vi "cam take photo-box.vi"(7 "error in":errorcluster) -> (20 "Image Out":T2(plugin-control), 22 "Session Out":T1, 27 "error out":errorcluster)   [LabVIEW 2019]
doc: "Creates, and edits acquisitions using the NI Vision Acquisition Express VI.\n\nThe NI Vision Acquisition Wizard is launched by placing the Express VI on the block diagram. Select an acquisition source and configure an acquisition using NI-IMAQ, NI-IMAQdx, or simulate an acquisition by reading an AVI or image files from a folder. After an acquisition is configured, select controls and indicators to be able to programmatically set in LabVIEW. Double-click the Vision Acquisition Express VI to edit the acquisition.\n\nNote: Any images created by the Express VI need to be disposed after use. Use the IMAQ Dispose.vi to cleanup the images output by the Express VI when they are no longer needed."
uses:
  <vilib>/userDefined/High Color/IMAQdx.ctl
  <vilib>/vision/driver/NI_Vision_Acquisition_Software.lvlib
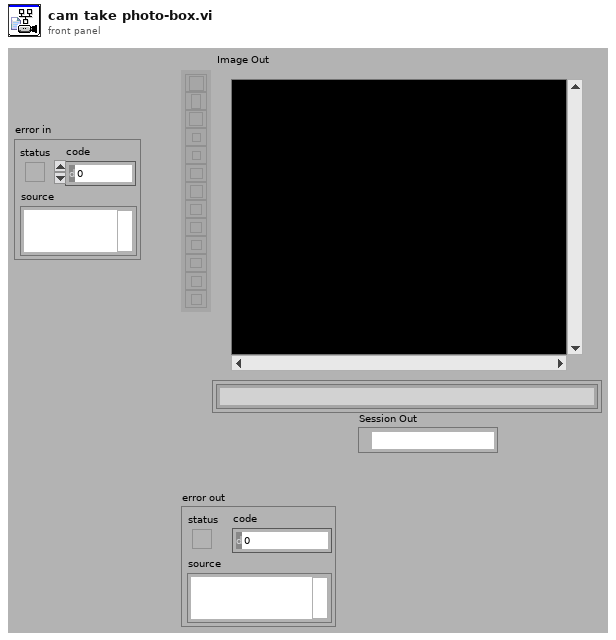
[diagram p1: front panel]
types:
  T1 = typedef "IMAQdx.ctl" = refnum<k21>
  T2 = typedef "IMAQ Image.ctl" = refnum<image>
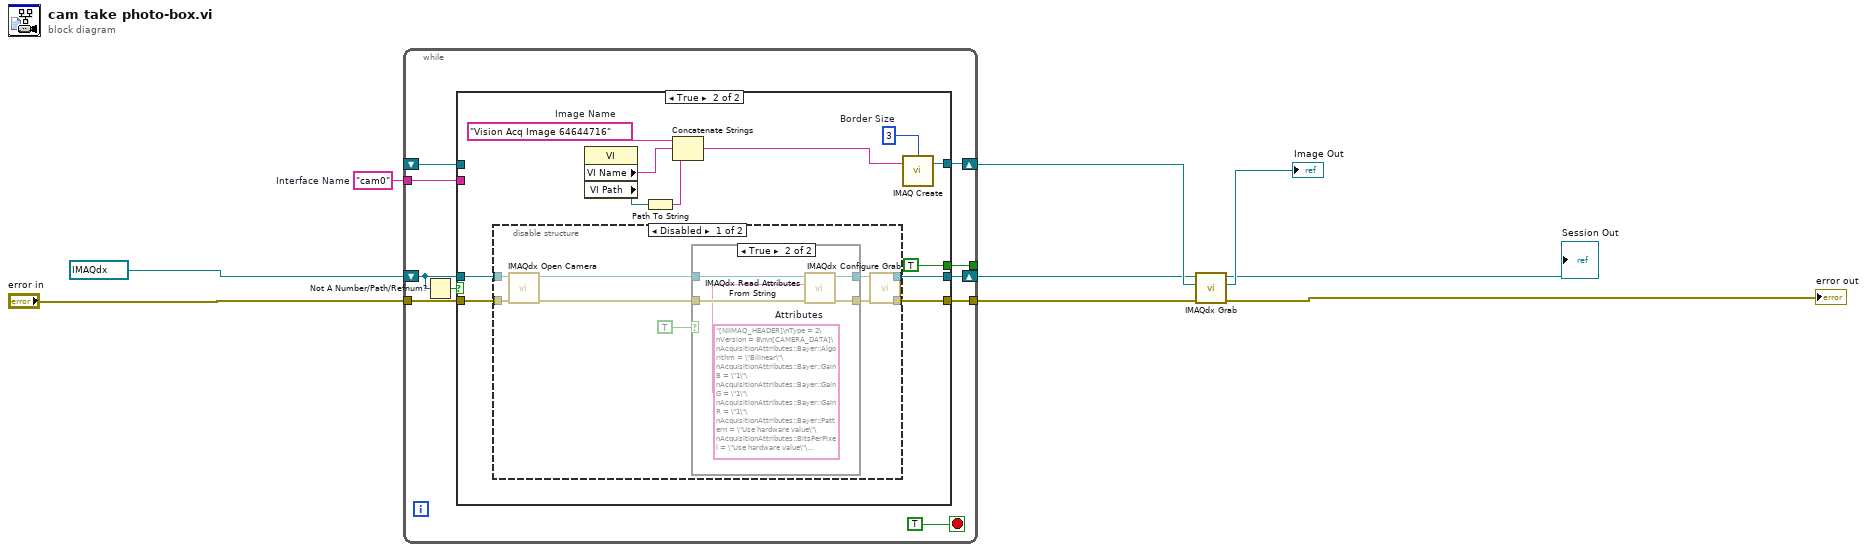
[diagram p0: block diagram]
diagram:
  w7 = "cam0"  # Interface Name
  n1 = while "While Loop_template0" {
    shift-right: [w19] -> w4
    shift-left: T1 "cam0" ("Session Out") -> [w12]
    tunnel: [w18] -> w8
    tunnel: "error in" -> [w17]
    shift-right: [w15] -> w5
    shift-left: _ -> [w14]
    tunnel: w7 -> [w13]
    tunnel: [w10] -> _
    stop <- TRUE ("_template0") stop-if-true
    n2 = Not A Number/Path/Refnum?(number/path/refnum=w12) -> (NaN/Path/Refnum?=w11:bool)
    n3 = case "Case Structure_template0" shown="True" w11 {
      tunnel: [w22 w33] -> w19
      tunnel: w12 -> [w22 w23]
      tunnel: [w21 w32] -> w18
      tunnel: w17 -> [w21 w34]
      tunnel: [w20 w31] -> w15
      tunnel: w14 -> [w20 _]
      tunnel: w13 -> [_ _]
      tunnel: [_ TRUE] -> w10
      frame False {
      }
      frame True {
        w24 = 3  # Border Size
        w26 = "Vision Acq Image 64644716"  # Image Name
        n4 = disable-structure shown="Disabled" {
          disable-tunnel: w34 -> [w43 w51]
          disable-tunnel: [w42 w52] -> w33
          disable-tunnel: [w41 w51] -> w32
          disable-tunnel: w23 -> [w35 w52]
          frame Disabled {
            n5 = call <vilib>:"IMAQdx Open Camera.vi"("error in"=w43, "Session In"=w35) -> ("error out"=w39:errorcluster, "Session Out"=w40:T1)  [unwired: 1 in, 7 out]
            n6 = case shown="True" TRUE ("Init Attributes") {
              tunnel: w40 -> [w45 w50]
              tunnel: w39 -> [w44 w49]
              tunnel: [w45 w47] -> w38
              tunnel: [w44 w46] -> w37
              frame False {
              }
              frame True {
                w48 = "[NIIMAQ_HEADER]\nType = 2\nVersion = 8\n\n[CAMERA_DATA]\nAcquisitionAttributes::Bayer::Algorithm = \"Bilinear\"\nAcquisitionAttributes::Bayer::GainB = \"1\"\nAcquisitionAttributes::Bayer::GainG = \"1\"\nAcquisitionAttributes::Bayer::GainR = \"1\"\nAcquisitionAttributes::Bayer::Pattern = \"Use hardware value\"\nAcquisitionAttributes::BitsPerPixel = \"Use hardware value\"\nAcquisitionAttributes::HardwareMaximumQueuedBufferCount = \"1000\"\nAcquisitionAttributes::HardwareRequeueBufferListThreshold = \"50\"\nAcquisitionAttributes::IgnoreFirstFrame = \"false\"\nAcquisitionAttributes::ImageDecoderCopyMode = \"Auto\"\nAcquisitionAttributes::OutputImageType = \"Auto\"\nAcquisitionAttributes::OverwriteMode = \"Get Newest\"\nAcquisitionAttributes::PixelSignedness = \"Use hardware value\"\nAcquisitionAttributes::ReceiveTimestampMode = \"None\"\nAcquisitionAttributes::ShiftPixelBits = \"false\"\nAcquisitionAttributes::SwapPixelBytes = \"false\"\nAcquisitionAttributes::Timeout = \"5000\"\nAcquisitionAttributes::VideoMode = \"160 x 120 YUY 2 30.00 fps\"\nCameraAttributes::BacklightCompensation::Mode = \"Manual\"\nCameraAttributes::BacklightCompensation::Value = \"0\"\nCameraAttributes::Brightness::Mode = \"Manual\"\nCameraAttributes::Brightness::Value = \"133\"\nCameraAttributes::Contrast::Mode = \"Manual\"\nCameraAttributes::Contrast::Value = \"5\"\nCameraAttributes::Exposure::Mode = \"AutoAperaturePriority\"\nCameraAttributes::Focus::Mode = \"Auto\"\nCameraAttributes::Pan::Mode = \"Manual\"\nCameraAttributes::Pan::Value = \"0\"\nCameraAttributes::PowerLineFrequency::Mode = \"60Hz\"\nCameraAttributes::Saturation::Mode = \"Manual\"\nCameraAttributes::Saturation::Value = \"83\"\nCameraAttributes::Sharpness::Mode = \"Manual\"\nCameraAttributes::Sharpness::Value = \"25\"\nCameraAttributes::Tilt::Mode = \"Manual\"\nCameraAttributes::Tilt::Value = \"0\"\nCameraAttributes::WhiteBalance::Mode = \"Auto\"\nCameraAttributes::Zoom::Mode = \"Manual\"\nCameraAttributes::Zoom::Value = \"0\"\n"  # Attributes
                n7 = call <vilib>:"IMAQdx Read Attributes From String.vi"("error in"=w49, "Attributes String In"=w48, "Session In"=w50) -> ("error out"=w46:errorcluster, "Session Out"=w47:T1)  [unwired: 7 out]
              }
            }
            n8 = call <vilib>:"IMAQdx Configure Grab.vi"("error in"=w37, "Session In"=w38) -> ("error out"=w41:errorcluster, "Session Out"=w42:T1)  [unwired: 1 in, 7 out]
          }
          frame Enabled {
          }
        }
        n9 = property class="VI"() -> ("VI Name"=w29:string, "VI Path"=w30:path)  [unwired: 2 in, 2 out]
        n10 = Path To String(path=w30) -> (string=w28:string)
        n11 = Concatenate Strings(w26, w29, w28) -> (w27:string)
        n12 = call "IMAQ Create"("Border Size"=w24, "Image Name"=w27) -> ("New Image"=w31:T2)  [unwired: 2 in, 2 out]
      }
    }
  }
  n13 = call <vilib>:"IMAQdx Grab.vi"("error in"=w8, "Image In"=w5, "Session In"=w4) -> ("error out"=→"error out":errorcluster, "Image Out"=→"Image Out":T2, "Session Out"=→"Session Out":T1)  [unwired: 1 in, 5 out]
